vi "Add Update Key.vi"(8 "error in":errorcluster, 9 "Value":string, 10 "Key":string, 11 "Config in":refnum<class "Config.lvclass">) -> (0 "error out":errorcluster, 3 "Config out":refnum<class "Config.lvclass">)   [LabVIEW 2023, in "Config.lvlib" / "Config.lvclass"]
uses:
  Config.lvclass
  Config.lvclass/Config.ctl
  <vilib>/Utility/config.llb/Write Key (String).vi
  <vilib>/Utility/config.llb/NI_LVConfig.lvlib
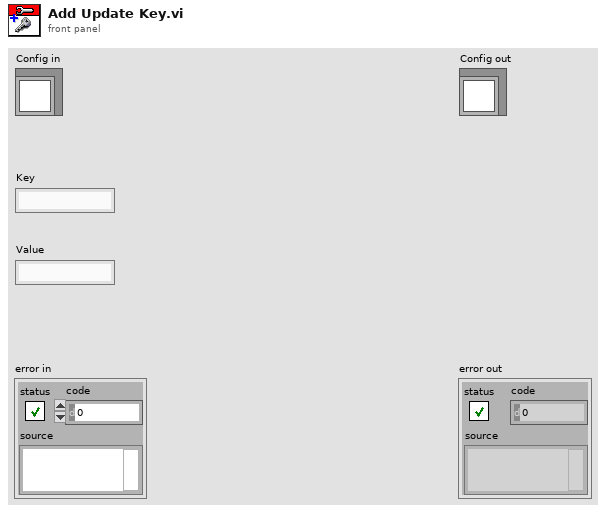
[diagram p1: front panel]
types:
  T1 = typedef "NI_LVConfig.lvlib/Config Data RefNum.ctl" = refnum<k1>
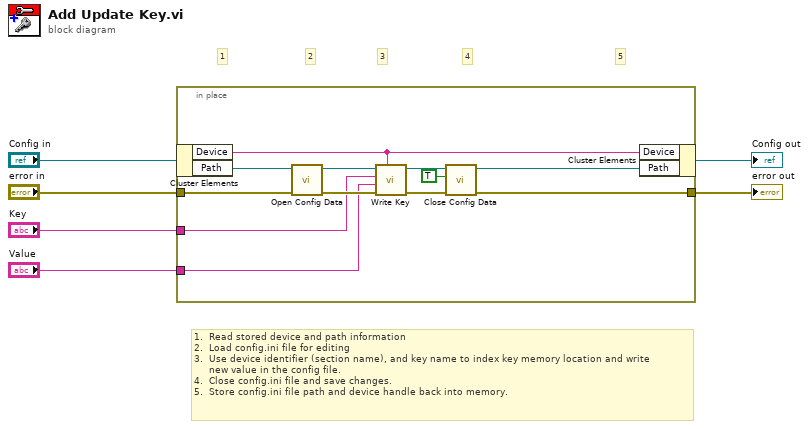
[diagram p0: block diagram]
diagram:
  # "1.  Read stored device and path information\n2.  Load config.ini file for editing\n3.  Use device identifier (section name), and key name to index key memory location and write \n     new value in the config file.\n4.  Close config.ini file and save changes.\n5.  Store config.ini file path and device handle back into memory."
  # "5"
  # "4"
  # "3"
  # "2"
  # "1"
  n1 = in-place {
    in-place-border: [w11] -> w5
    in-place-border: "error in" -> [w10]
    in-place-border: "Key" -> [w9]
    in-place-border: "Value" -> [w8]
    n2 = in-place-cluster #1("Config in") -> ("Device"=w16:string, "Path"=w15:path)
    n3 = call <vilib>:"Open Config Data.vi"("error in (no error)"=w10, "configuration file path"=w15) -> ("error out"=w13:errorcluster, "refnum"=w18:T1)  [unwired: 7 in, 1 out]
    n4 = call-poly <vilib>:"Write Key.vi"("section"=w16, "error in (no error)"=w13, "value"=w8, "key"=w9, "refnum"=w18) -> ("error out"=w12:errorcluster, "refnum out"=w17:T1)  [unwired: 4 in, 1 out]
    n5 = call <vilib>:"Close Config Data.vi"("error in (no error)"=w12, "write file if changed (T)"=TRUE, "refnum"=w17) -> ("error out"=w11:errorcluster, "file path"=w14:path)  [unwired: 7 in]
    n6 = in-place-cluster #1("Device"=w16, "Path"=w14) -> (→"Config out":refnum<class "Config.lvclass">)
  }
  "error out" <- w5
